vi "Create TDMS File.vi"(8 "error in (no error)":errorcluster, 9 "TDMS File Attribute":cluster{"Name":string, "Value":string}[](array[cluster]), 10 "File Path":path, 11 "TDMS-Actor in":refnum<class "TDMS-Actor.lvclass">) -> (0 "error out":errorcluster, 3 "TDMS-Actor out":refnum<class "TDMS-Actor.lvclass">)   [LabVIEW 2017, in "BNT_TDMS.lvlib" / "TDMS-Actor.lvclass"]
doc: "Create TDMs-File as specified, in base path if relative, or in default directory with Date-Time.tdms as name."
uses:
  TDMS-Actor.lvclass
  TDMS-Actor.lvclass/TDMS-Actor.ctl
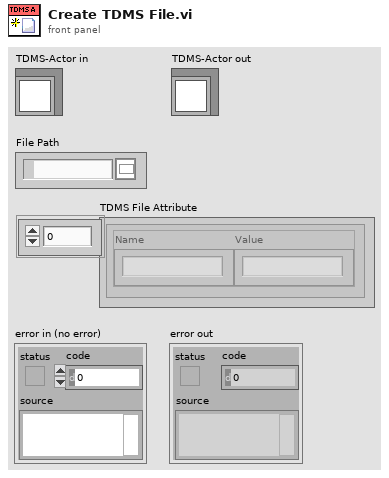
[diagram p1: front panel]
types:
  T1 = enum16{"open", "open or create", "create or replace", "create", "open (read-only)"}
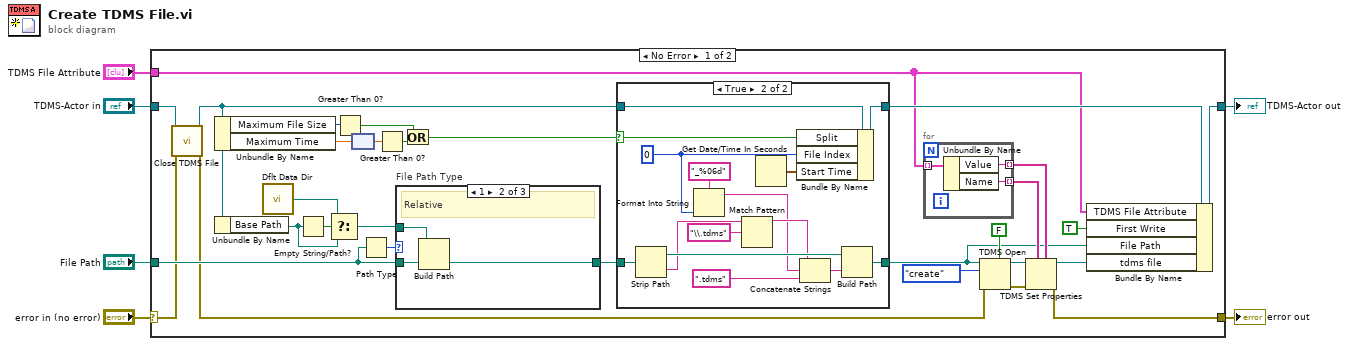
[diagram p0: block diagram]
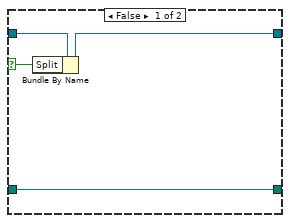
[diagram p2: hidden frame]
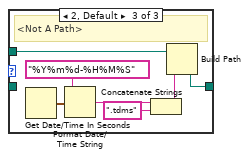
[diagram p4: hidden frame]
diagram:
  n1 = case shown="No Error" "error in (no error)" {
    selector: "error in (no error)" -> [w20 w71]
    tunnel: [w24 w71] -> w5
    tunnel: [w28 w70] -> w3
    tunnel: "TDMS-Actor in" -> [w21 w70]
    tunnel: "File Path" -> [w32 _]
    tunnel: "TDMS File Attribute" -> [w7 _]
    frame No Error {
      n2 = call "Close TDMS File.vi"("error in (no error)"=w20, "TDMS-Actor in"=w21) -> ("error out"=w19:errorcluster, "TDMS-Actor out"=w17:refnum<class "TDMS-Actor.lvclass">)  [unwired: 8 in]
      n3 = Unbundle By Name(w17) -> ("Maximum File Size"=w15:i64, "Maximum Time"=w14:dbl[unit])
      n4 = Unbundle By Name(w17) -> ("Base Path"=w34:path)
      n5 = call <vilib>:"Dflt Data Dir.vi"() -> ("App:Default Data Directory"=w35:path)
      n6 = Empty String/Path?(string/path=w34) -> (empty?=w36:bool)
      n7 = Select(t=w35, s=w36, f=w34) -> (s? t:f=w31:path)
      n8 = Greater Than 0?(x=w15) -> (x > 0?=w11:bool)
      n9 = node(w14) -> (w13:dbl)
      n10 = Path Type(1:w32) -> (0:w33:i16)
      n11 = Greater Than 0?(x=w13) -> (x > 0?=w12:bool)
      n12 = case "File Path Type" shown="1" w33 {
        tunnel: w32 -> [w59 w62 _]
        tunnel: [w59 w60 w67] -> w9
        tunnel: w31 -> [_ w61 w69]
        frame 0 {
          # "Absolute"
        }
        frame 1 {
          # "Relative"
          n13 = Build Path(base path=w61, name or relative path=w62) -> (appended path=w60:path)
        }
        frame 2, Default {
          # "<Not A Path>"
          n14 = Get Date/Time In Seconds() -> (seconds since 1Jan1904=w68:timestamp)
          n15 = Format Date/Time String(time format string (%c)="%Y%m%d-%H%M%S", seconds (now)=w68) -> (date/time string=w65:string)  [unwired: 1 in]
          n16 = Concatenate Strings(w65, ".tdms" ("string")) -> (w63:string)
          n17 = Build Path(base path=w69, name or relative path=w63) -> (appended path=w67:path)
        }
      }
      n18 = Or(x=w11, y=w12) -> (x .or. y?=w8:bool)
      n19 = case shown="True" w8 {
        selector: w8 -> [w37 w53]
        tunnel: w17 -> [w39 w55]
        tunnel: [w38 w54] -> w16
        tunnel: [w40 w49] -> w10
        tunnel: w9 -> [w40 w52]
        frame False {
          n20 = Bundle By Name(cluster=w39, "Split"=w37) -> (w38:refnum<class "TDMS-Actor.lvclass">)
        }
        frame True {
          w44 = 0 ("File Index")
          n21 = Strip Path(path=w52) -> (stripped path=w50:path, name=w48:string)
          n22 = Format Into String(format string="_%06d", w44) -> (resulting string=w42:string)  [unwired: 2 in, 1 out]
          n23 = Match Pattern(string=w48, regular expression="\\.tdms") -> (before substring=w46:string)  [unwired: 1 in, 3 out]
          n24 = Get Date/Time In Seconds() -> (seconds since 1Jan1904=w41:timestamp)
          n25 = Bundle By Name(cluster=w55, "Split"=w53, "File Index"=w44, "Start Time"=w41) -> (w54:refnum<class "TDMS-Actor.lvclass">)
          n26 = Concatenate Strings(w46, w42, ".tdms" ("string")) -> (w51:string)
          n27 = Build Path(base path=w50, name or relative path=w51) -> (appended path=w49:path)
        }
      }
      n28 = for {
        tunnel: w7 -> [w58] mode=indexing
        tunnel: [w57] -> w23 mode=indexing
        tunnel: [w56] -> w22 mode=indexing
        n29 = Unbundle By Name(w58) -> ("Value"=w56:string, "Name"=w57:string)
      }
      n30 = TDMS Open(5:FALSE ("create index file? (T)"), 8:w19, 10:T1."create" ("operation (0:open)"), 11:w10) -> (0:w25:errorcluster, 3:w27:refnum<k34>)  [unwired: 3 in]
      n31 = TDMS Set Properties(5:w22, 7:w23, 8:w25, 11:w27) -> (0:w24:errorcluster, 3:w26:refnum<k34>)  [unwired: 2 in, 2 out]
      n32 = Bundle By Name(cluster=w16, "TDMS File Attribute"=w7, "First Write"=TRUE, "File Path"=w10, "tdms file"=w26) -> (w28:refnum<class "TDMS-Actor.lvclass">)
    }
    frame Error {
    }
  }
  "error out" <- w5
  "TDMS-Actor out" <- w3
